vi "DAQ Digital Code Scan.vi"(8 "error in (no error)":errorcluster, 11 "DAQ Digital Code Scan.lvclass":refnum<class "DAQ Digital Code Scan.lvclass">) -> (0 "error out":errorcluster, 3 "DAQ Digital Code Scan.lvclass 2":refnum<class "DAQ Digital Code Scan.lvclass">)   [LabVIEW 2012, in "DAQ Digital Code Scan.lvclass"]
uses:
  DAQ Digital Code Scan.lvclass
  DAQ Digital Code Scan.lvclass/DAQ Digital Code Scan.ctl
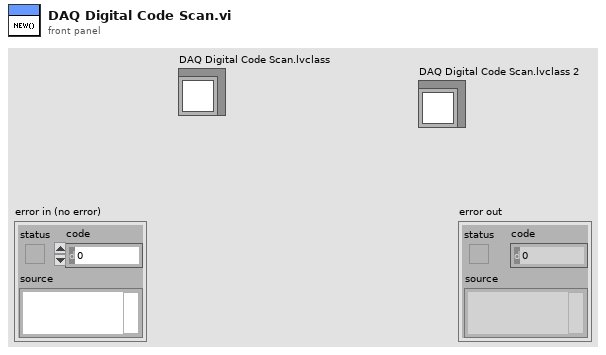
[diagram p1: front panel]
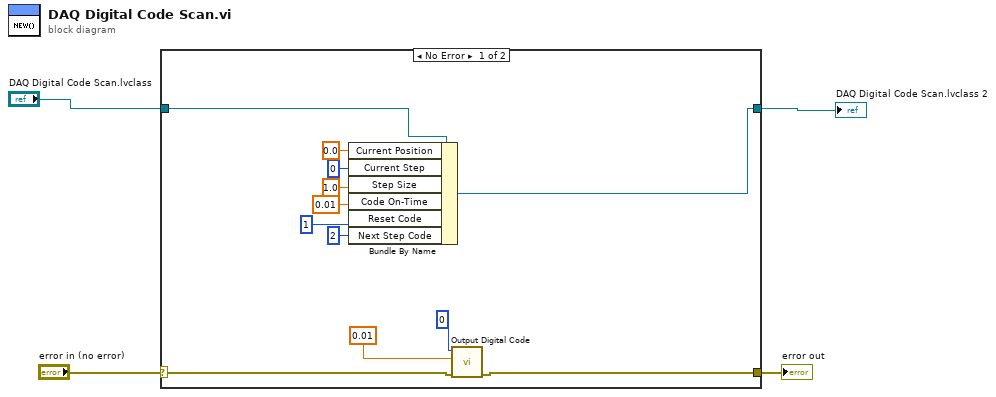
[diagram p0: block diagram]
diagram:
  n1 = case shown="No Error" "error in (no error)" {
    selector: "error in (no error)" -> [w11 w18]
    tunnel: [w10 w18] -> w3
    tunnel: [w13 w17] -> w1
    tunnel: "DAQ Digital Code Scan.lvclass" -> [w16 w17]
    frame No Error {
      n2 = Bundle By Name(cluster=w16, "Current Position"=0.0, "Current Step"=u32 0, "Step Size"=1.0, "Code On-Time"=0.01, "Reset Code"=i8 1, "Next Step Code"=i8 2) -> (w13:refnum<class "DAQ Digital Code Scan.lvclass">)
      n3 = call "Output Digital Code.vi"("error in (no error)"=w11, "Pulse Time"=0.01, "Input"=i8 0) -> ("error out"=w10:errorcluster)  [unwired: 6 in]
    }
    frame Error {
    }
  }
  "error out" <- w3
  "DAQ Digital Code Scan.lvclass 2" <- w1
